vi "InitialiseOLED.vi"(8 "error in (no error)":errorcluster) -> (0 "error out":errorcluster, 3 "Messages":string[](array[string]))   [LabVIEW 2024, in "OLEDI2CMessageGenerator.lvlib"]
uses:
  OLEDI2CMessageGenerator.lvlib
panel:
  # "Input"
  # "Output"
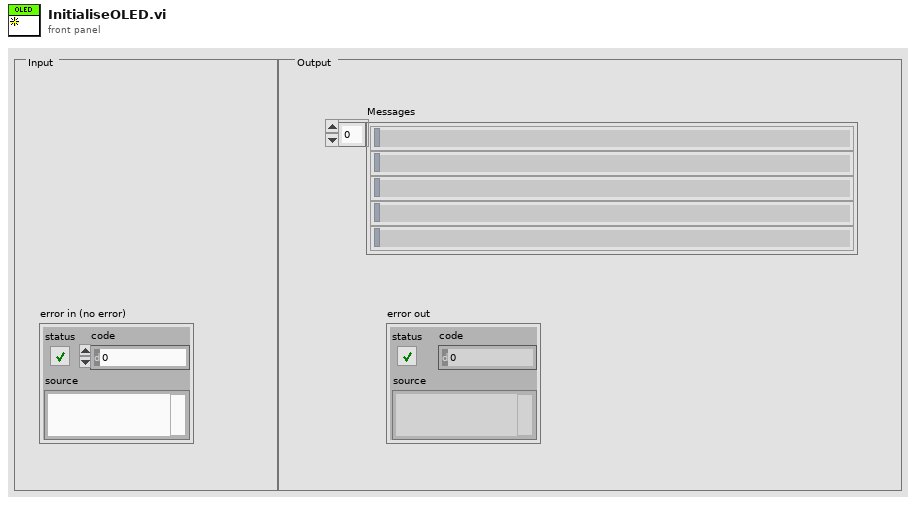
[diagram p1: front panel]
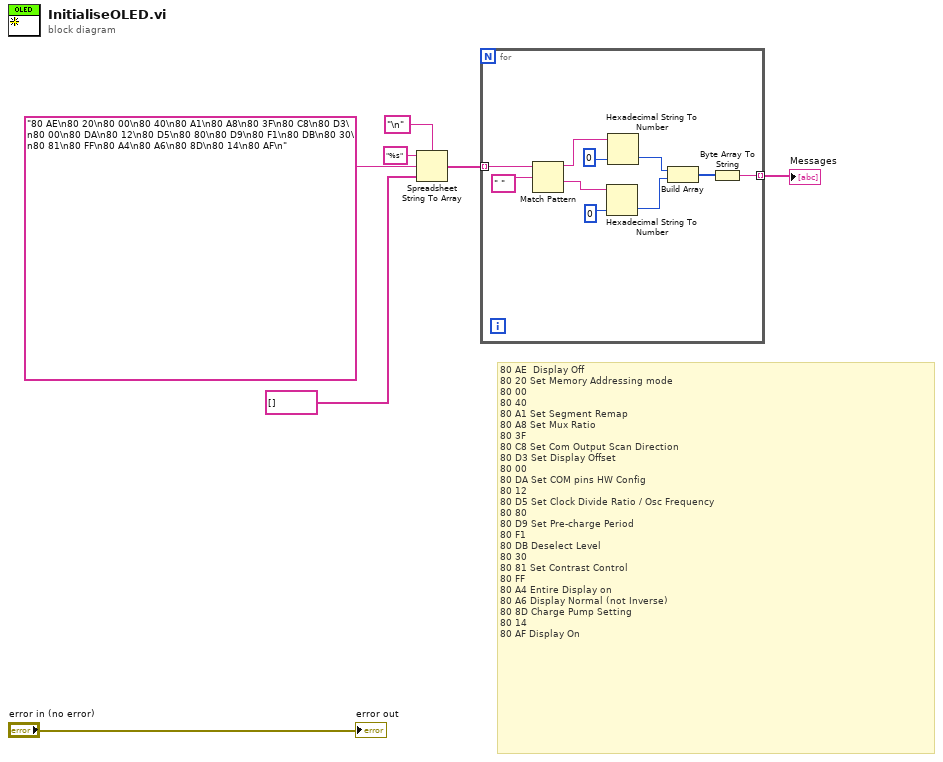
[diagram p0: block diagram]
diagram:
  # "80 AE  Display Off\n80 20 Set Memory Addressing mode\n80 00 \n80 40\n80 A1 Set Segment Remap\n80 A8 Set Mux Ratio\n80 3F\n80 C8 Set Com Output Scan Direction\n80 D3 Set Display Offset\n80 00\n80 DA Set COM pins HW Config\n80 12\n80 D5 Set Clock Divide Ratio / Osc Frequency\n80 80\n80 D9 Set Pre-charge Period\n80 F1\n80 DB Deselect Level\n80 30\n80 81 Set Contrast Control\n80 FF\n80 A4 Entire Display on\n80 A6 Display Normal (not Inverse)\n80 8D Charge Pump Setting\n80 14\n80 AF Display On"
  n1 = Spreadsheet String To Array(delimiter (Tab)="\n", format string="%s", spreadsheet string="80 AE\n80 20\n80 00\n80 40\n80 A1\n80 A8\n80 3F\n80 C8\n80 D3\n80 00\n80 DA\n80 12\n80 D5\n80 80\n80 D9\n80 F1\n80 DB\n80 30\n80 81\n80 FF\n80 A4\n80 A6\n80 8D\n80 14\n80 AF\n", array type (2D Dbl)=string[] []) -> (array=w2:string[])
  n2 = for {
    tunnel: w2 -> [w14] mode=indexing
    tunnel: [w10] -> w1 mode=indexing
    n3 = Match Pattern(string=w14, regular expression=" " ("delimiter (Tab)")) -> (before substring=w16:string, after substring=w15:string)  [unwired: 1 in, 2 out]
    n4 = Hexadecimal String To Number(string=w15, default (0uL)=u8 0) -> (number=w12:u8)  [unwired: 1 in, 1 out]
    n5 = Hexadecimal String To Number(string=w16, default (0uL)=u8 0) -> (number=w13:u8)  [unwired: 1 in, 1 out]
    n6 = Build Array(w13, w12) -> (w11:u8[])
    n7 = Byte Array To String(unsigned byte array=w11) -> (string=w10:string)
  }
  "Messages" <- w1
  "error out" <- "error in (no error)"
